vi "testNetworkCam.vi"() -> ()   [LabVIEW 2009, in "run.lvlib"]
uses:
  run.lvlib
  Tools/Filing/FileSystem/FileSystem.lvclass
  Tools/CameraSettings/CamaraSettings.lvclass
  HWController/Network Controllers/NetworkCamera/NetworkCamera.lvclass
  Tools/Filing/FileNeologist/FileNeologist.lvclass
panel:
  in  "stop 2":bool
  out "stopped 2":bool
  in  "run image viewer":bool
  in  "stop":bool
  out "stopped":bool
  in  "number":i32=-1
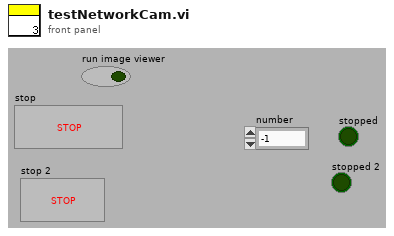
[diagram p1: front panel]
types:
  T1 = enum32{"Invalid", "Standard", "Closed", "Hidden", "Minimized", "Maximized"}
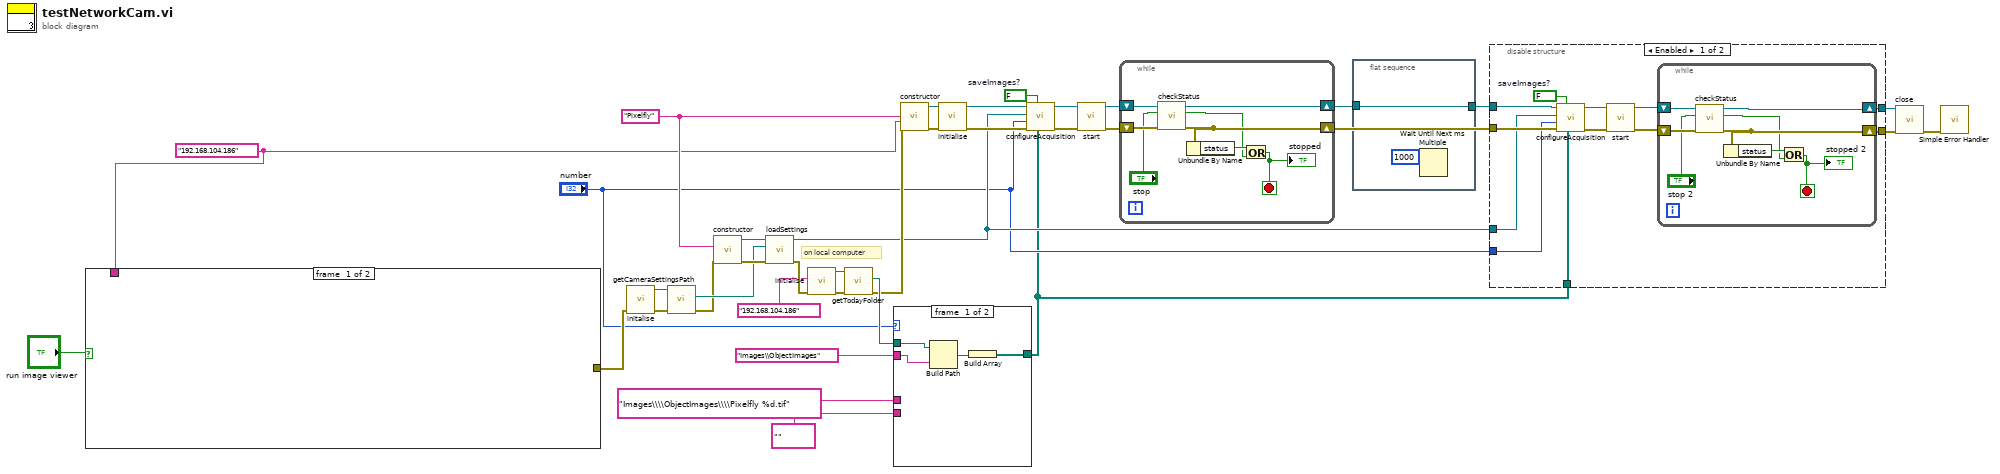
[diagram p0: block diagram]
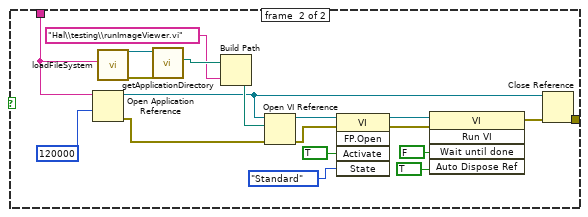
[diagram p3: hidden frame]
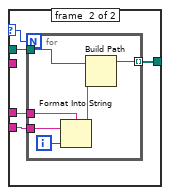
[diagram p4: hidden frame]
diagram:
  w19 = FALSE  # saveImages?
  w11 = "192.168.104.186"
  w16 = "Pixelfly"
  # "on local computer"
  n1 = case shown="True" "run image viewer" {
    tunnel: w11 -> [_ w56]
    tunnel: [_ w55] -> w10
    frame #0 {
    }
    frame #1 {
      n2 = Open Application Reference(9:120000 ("timeout ms (60000)"), 11:w56) -> (0:w54:errorcluster, 3:w45:refnum<vi>)  [unwired: 2 in]
      n3 = call "loadFileSystem.vi"("computer name"=w56) -> ("error out"=w52:errorcluster, "FileSystem out"=w53:refnum<class "FileSystem.lvclass">)  [unwired: 9 in]
      n4 = call-dynamic "getApplicationDirectory.vi"("error in (no error)"=w52, "FileSystem.lvclass in"=w53) -> ("ApplicationDirectory"=w51:path)  [unwired: 7 in, 2 out]
      n5 = Build Path(base path=w51, name or relative path="Hal\\testing\\runImageViewer.vi") -> (appended path=w49:path)
      n6 = Open VI Reference(application reference (local)=w45, vi path=w49, error in (no error)=w54) -> (vi reference=w48:refnum<vi>, error out=w39:errorcluster)  [unwired: 3 in]
      n7 = invoke class="VI" method="FP.Open"(reference=w48, error in=w39, "Activate"=TRUE ("Activate?"), "State"=T1."Standard") -> (reference out=w42:refnum<vi>, error out=w38:errorcluster)  [unwired: 1 in, 3 out]
      n8 = invoke class="VI" method="Run VI"(reference=w42, error in=w38, "Wait until done"=FALSE, "Auto Dispose Ref"=TRUE ("Auto Dispose Reference")) -> (error out=w44:errorcluster)  [unwired: 1 in, 4 out]
      n9 = Close Reference(reference=w45, error in (no error)=w44) -> (error out=w55:errorcluster)
    }
  }
  n10 = call "initalise.vi"("error in (no error)"=w10) -> ("error out"=w32:errorcluster, "FileSystem out"=w33:refnum<class "FileSystem.lvclass">)  [unwired: 9 in]
  n11 = call-dynamic "getCameraSettingsPath.vi"("error in (no error)"=w32, "FileSystem.lvclass in"=w33) -> ("error out"=w30:errorcluster, "CameraSettingsPath"=w31:path)  [unwired: 7 in, 1 out]
  n12 = call "constructor.vi"("error in (no error)"=w30, "camera settings"=w16) -> ("error out"=w34:errorcluster, "CamaraSettings out"=w35:refnum<class "CamaraSettings.lvclass">)  [unwired: 8 in]
  n13 = call-dynamic "loadSettings.vi"("error in (no error)"=w34, "Path"=w31, "CamaraSettings in"=w35) -> ("error out"=w29:errorcluster, "CamaraSettings out"=w7:refnum<class "CamaraSettings.lvclass">)  [unwired: 7 in]
  n14 = call "initialise.vi"("error in (no error)"=w29, "computer name"="192.168.104.186") -> ("error out"=w27:errorcluster, "FileNeologist out"=w28:refnum<class "FileNeologist.lvclass">)  [unwired: 8 in]
  n15 = call "getTodayFolder.vi"("error in (no error)"=w27, "FileNeologist in"=w28) -> ("error out"=w20:errorcluster, "todayFolder"=w26:path)  [unwired: 7 in, 1 out]
  n16 = case shown="1, Default" "number" {
    selector: "number" -> [_ w62]
    tunnel: w26 -> [w59 w65]
    tunnel: [w60 w64] -> w5
    tunnel: "Images\\\\ObjectImages\\\\Pixelfly %d.tif" -> [_ w63]
    tunnel: "" -> [_ w61]
    tunnel: "Images\\ObjectImages" -> [w58 _]
    frame #0 {
      n17 = Build Path(base path=w59, name or relative path=w58) -> (appended path=w57:path)
      n18 = Build Array(w57) -> (w60:path[])
    }
    frame #1 {
      n19 = for {
        N: w62 -> [_]
        tunnel: w65 -> [w71]
        tunnel: [w70] -> w64 mode=indexing
        tunnel: w63 -> [w68]
        tunnel: w61 -> [w66]
        i -> [w69]
        n20 = Format Into String(format string=w68, initial string=w66, w69) -> (resulting string=w67:string)  [unwired: 1 in, 1 out]
        n21 = Build Path(base path=w71, name or relative path=w67) -> (appended path=w70:path)
      }
    }
  }
  n22 = call "constructor.vi"("error in (no error)"=w20, "machine name"=w11, "Camera"=w16) -> ("error out"=w36:errorcluster, "NetworkCamera out"=w37:refnum<class "NetworkCamera.lvclass">)  [unwired: 7 in]
  n23 = call-dynamic "initialise.vi"("error in (no error)"=w36, "NetworkCamera in"=w37) -> ("error out"=w21:errorcluster, "NetworkCamera out"=w22:refnum<class "NetworkCamera.lvclass">)  [unwired: 8 in]
  n24 = call-dynamic "configureAcquisition.vi"("imagePaths"=w5, "saveImages?"=w19, "error in (no error)"=w21, "number of Images"="number", "CamaraSettings"=w7, "NetworkCamera in"=w22) -> ("error out"=w17:errorcluster, "NetworkCamera out"=w18:refnum<class "NetworkCamera.lvclass">)  [unwired: 4 in]
  n25 = call-dynamic "start.vi"("error in (no error)"=w17, "NetworkCamera in"=w18) -> ("error out"=w14:errorcluster, "NetworkCamera out"=w15:refnum<class "NetworkCamera.lvclass">)  [unwired: 8 in]
  n26 = while {
    shift-right: [w76] -> w1
    shift-left: w15 -> [w77]
    shift-right: [w74] -> w8
    shift-left: w14 -> [w75]
    stop <- w78 stop-if-true
    n27 = call-dynamic "checkStatus.vi"("error in (no error)"=w75, "stop"="stop", "NetworkCamera in"=w77) -> ("error out"=w74:errorcluster, "stopped?"=w73:bool, "NetworkCamera out"=w76:refnum<class "NetworkCamera.lvclass">)  [unwired: 6 in]
    n28 = Unbundle By Name(w74) -> ("status"=w79:bool)
    n29 = Or(x=w79, y=w73) -> (x .or. y?=w78:bool)
    "stopped" <- w78
  }
  n30 = flat-sequence {
    tunnel: [w81] -> w2
    tunnel: w1 -> [w81]
    frame #0 {
      n31 = Wait Until Next ms Multiple(millisecond multiple=1000) -> ()  [unwired: 1 out]
    }
  }
  n32 = disable-structure shown="Enabled" {
    disable-tunnel: w8 -> [w93 w102]
    disable-tunnel: w7 -> [w92 _]
    disable-tunnel: "number" -> [w91 _]
    disable-tunnel: w5 -> [w90 _]
    disable-tunnel: [w89 w103] -> w4
    disable-tunnel: [w88 w102] -> w3
    disable-tunnel: w2 -> [w87 w103]
    frame #0 {
      w86 = FALSE  # saveImages?
      n33 = call-dynamic "configureAcquisition.vi"("imagePaths"=w90, "saveImages?"=w86, "error in (no error)"=w93, "number of Images"=w91, "CamaraSettings"=w92, "NetworkCamera in"=w87) -> ("error out"=w84:errorcluster, "NetworkCamera out"=w85:refnum<class "NetworkCamera.lvclass">)  [unwired: 4 in]
      n34 = call-dynamic "start.vi"("error in (no error)"=w84, "NetworkCamera in"=w85) -> ("error out"=w82:errorcluster, "NetworkCamera out"=w83:refnum<class "NetworkCamera.lvclass">)  [unwired: 8 in]
      n35 = while {
        shift-right: [w98] -> w89
        shift-left: w83 -> [w99]
        shift-right: [w96] -> w88
        shift-left: w82 -> [w97]
        stop <- w100 stop-if-true
        n36 = call-dynamic "checkStatus.vi"("error in (no error)"=w97, "stop"="stop 2", "NetworkCamera in"=w99) -> ("error out"=w96:errorcluster, "stopped?"=w95:bool, "NetworkCamera out"=w98:refnum<class "NetworkCamera.lvclass">)  [unwired: 6 in]
        n37 = Unbundle By Name(w96) -> ("status"=w101:bool)
        n38 = Or(x=w101, y=w95) -> (x .or. y?=w100:bool)
        "stopped 2" <- w100
      }
    }
    frame #1 {
    }
  }
  n39 = call-dynamic "close.vi"("error in (no error)"=w3, "NetworkCamera in"=w4) -> ("error out"=w13:errorcluster)  [unwired: 9 in]
  n40 = call <vilib>:"Simple Error Handler.vi"("error in (no error)"=w13) -> ()  [unwired: 4 in, 5 out]
